vi "Iterate.vi"(10 "Iterate":i32) -> (2 "Msg Strategy":refnum<class "Msg Strategy.lvclass">)   [LabVIEW 2021, in "Hello World Event.lvlib" / "Iterate Msg Strategy.lvlib"]
uses:
  Iterate Msg Strategy.lvlib
  <vilib>/Nathan Davis/jettl/jettl/Msg Strategy/Msg Strategy.lvclass
  Iterate Msg Strategy/Iterate Msg Strategy.lvclass
  C:/Program Files/National Instruments/LabVIEW 2021/vi.lib/Nathan Davis/jettl/jettl/Msg Strategy/Msg Strategy.lvclass
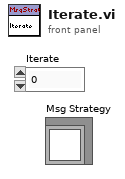
[diagram p1: front panel]
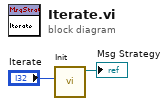
[diagram p0: block diagram]
diagram:
  n1 = call "Init.vi"("Iterate"="Iterate") -> ("Iterate Msg Strategy out"=→"Msg Strategy":refnum<class "Iterate Msg Strategy.lvclass">)  [unwired: 10 in]
